vi "RSZVB Wait For OPC.vi"(8 "error in (no error)":errorcluster {"code" format="%.0x"}, 9 "Timeout (300000 ms)":u32=300000, 10 "Command":string="*OPC?", 11 "VISA session":refnum<visa-resource-name>) -> (0 "error out":errorcluster {"code" format="%.0x"}, 2 "Read Buffer":string, 3 "dup VISA session":refnum<visa-resource-name>)   [LabVIEW 2015]
doc: "This VI send a command to the instrument and waits for the response."
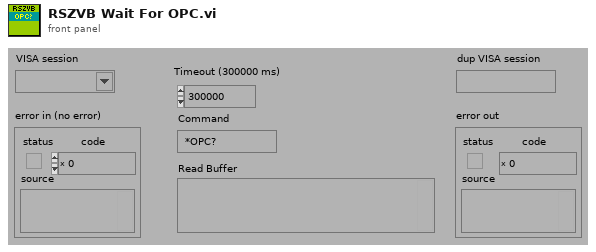
[diagram p1: front panel]
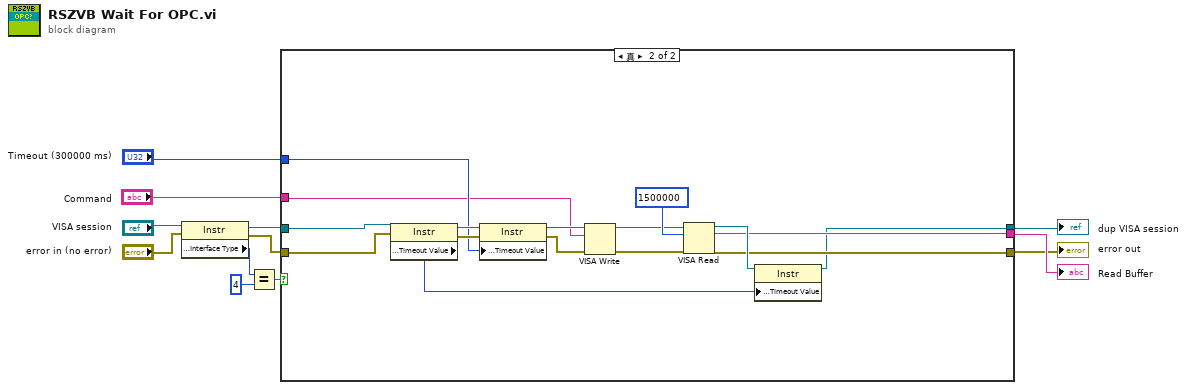
[diagram p0: block diagram]
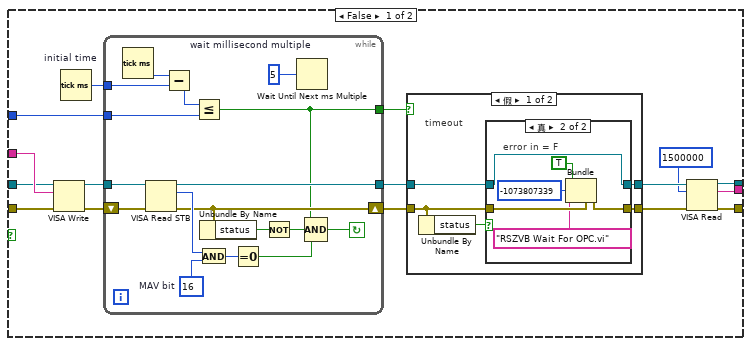
[diagram p2: hidden frame]
diagram:
  n1 = property class="Instr"(reference="VISA session", error in="error in (no error)") -> (reference out=w6:refnum<visa-resource-name>, error out=w5:errorcluster, "Interface Information:Interface Type"=w10:u16)
  n2 = Equal?(x=w10, y=u16 4) -> (x = y?=w4:bool)
  n3 = case shown="真" w4 {
    tunnel: [w18 w66] -> w3
    tunnel: "Timeout (300000 ms)" -> [w24 w65]
    tunnel: "Command" -> [w23 w64]
    tunnel: w5 -> [w22 w67]
    tunnel: w6 -> [w21 w61]
    tunnel: [w15 w62] -> w2
    tunnel: [w14 w63] -> w11
    frame False {
      n4 = VISA Write(VISA resource name=w21, write buffer=w23, error in (no error)=w22) -> (VISA resource name out=w19:refnum<visa-resource-name>, error out=w20:errorcluster)  [unwired: 1 out]
      n5 = Tick Count (ms) "initial time"() -> (millisecond timer value=w25:u32)
      n6 = while {
        tunnel: [w29] -> w26
        tunnel: w25 -> [w37]
        tunnel: w24 -> [w35]
        shift-left: w20 -> [w45]
        shift-right: [w34] -> w28
        tunnel: [w43] -> w27
        tunnel: w19 -> [w44]
        stop <- w31 continue-if-true
        w39 = u32 5  # wait millisecond multiple
        w41 = u16 16  # MAV bit
        n7 = Tick Count (ms)() -> (millisecond timer value=w38:u32)
        n8 = VISA Read STB(8:w45, 11:w44) -> (0:w34:errorcluster, 2:w42:u16, 3:w43:refnum<visa-resource-name>)
        n9 = Subtract(x=w38, y=w37) -> (x-y=w36:u32)
        n10 = Less Or Equal?(x=w36, y=w35) -> (x <= y?=w29:bool)
        n11 = And(x=w42, y=w41) -> (x .and. y?=w40:u16)
        n12 = Unbundle By Name(w34) -> ("status"=w33:bool)
        n13 = Equal To 0?(x=w40) -> (x = 0?=w30:bool)
        n14 = Not(x=w33) -> (.not. x?=w32:bool)
        n15 = Wait Until Next ms Multiple(millisecond multiple=w39) -> ()  [unwired: 1 out]
        n16 = Compound Arithmetic op=AND(w29, w32, w30) -> (w31:bool)
      }
      n17 = case shown="假" w26 {
        tunnel: w27 -> [w47 w60]
        tunnel: w28 -> [w49 w59]
        tunnel: [w48 w59] -> w17
        tunnel: [w46 w60] -> w16
        frame False {
          # "timeout"
          n18 = Unbundle By Name(w49) -> ("status"=w50:bool)
          n19 = case shown="真" w50 {
            tunnel: w49 -> [w52 w58]
            tunnel: [w52 w54] -> w48
            tunnel: w47 -> [w51 w53]
            tunnel: [w51 w53] -> w46
            frame False {
              # "error in = T"
            }
            frame True {
              # "error in = F"
              n20 = Bundle(cluster=w58, "status"=TRUE, "code"=-1073807339, "source"="RSZVB Wait For OPC.vi") -> (w54:errorcluster)
            }
          }
        }
        frame True {
          # "no timeout"
        }
      }
      n21 = VISA Read(VISA resource name=w16, byte count=u32 1500000 ("byte count (0)"), error in (no error)=w17) -> (VISA resource name out=w15:refnum<visa-resource-name>, read buffer=w14:string, error out=w18:errorcluster)  [unwired: 1 out]
    }
    frame True {
      n22 = property class="Instr"(reference=w61, error in=w67) -> (reference out=w76:refnum<visa-resource-name>, error out=w75:errorcluster, "General Settings:Timeout Value"=w72:u32)
      n23 = property class="Instr"(reference=w76, error in=w75, "General Settings:Timeout Value"=w65) -> (reference out=w74:refnum<visa-resource-name>, error out=w73:errorcluster)
      n24 = VISA Write(VISA resource name=w74, write buffer=w64, error in (no error)=w73) -> (VISA resource name out=w70:refnum<visa-resource-name>, error out=w69:errorcluster)  [unwired: 1 out]
      n25 = VISA Read(VISA resource name=w70, byte count=u32 1500000 ("byte count (0)"), error in (no error)=w69) -> (VISA resource name out=w68:refnum<visa-resource-name>, read buffer=w63:string, error out=w66:errorcluster)  [unwired: 1 out]
      n26 = property class="Instr"(reference=w68, "General Settings:Timeout Value"=w72) -> (reference out=w62:refnum<visa-resource-name>)  [unwired: 1 in, 1 out]
    }
  }
  "error out" <- w3
  "dup VISA session" <- w2
  "Read Buffer" <- w11
